vi "NewPort_PM_USB_CloseDevice(SubVI).vi"(8 "error in":errorcluster, 11 "reference In":refnum<k24>) -> (0 "error out":errorcluster)   [LabVIEW 2017]
uses:
  C:/Program Files (x86)/Newport/Newport USB Driver/Bin/UsbDllWrap.dll
  Program Files (x86)/Newport/Newport USB Driver/Bin/UsbDllWrap.dll
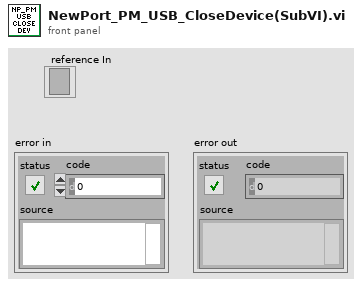
[diagram p1: front panel]
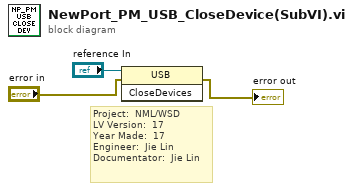
[diagram p0: block diagram]
diagram:
  # "Project:  NML/WSD \nLV Version:  17\nYear Made:  17\nEngineer:  Jie Lin\nDocumentator:  Jie Lin"
  n1 = invoke class="USB" method="CloseDevices"(reference="reference In", error in="error in") -> (error out=→"error out":errorcluster)  [unwired: 1 in, 2 out]
